vi "Write Y.vi"(8 "error in (no error)":errorcluster, 10 "Y":dbl[](array[numeric]), 11 "Y (1Ch) in":refnum<class "Y (1 Ch).lvclass">) -> (0 "error out":errorcluster, 3 "Y (1Ch) out":refnum<class "Y (1 Ch).lvclass">)   [LabVIEW 2017, in "Y (1 Ch).lvclass"]
uses:
  <vilib>/addons/_NISVFA/_Shared subVIs/Data Objects/Y (DBL)/Y (1 Ch).lvclass
  <vilib>/addons/_NISVFA/_Shared subVIs/Data Objects/Y (DBL)/Y (1 Ch).lvclass/Y (1 Ch).ctl
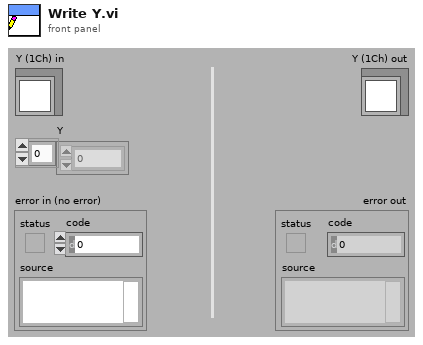
[diagram p1: front panel]
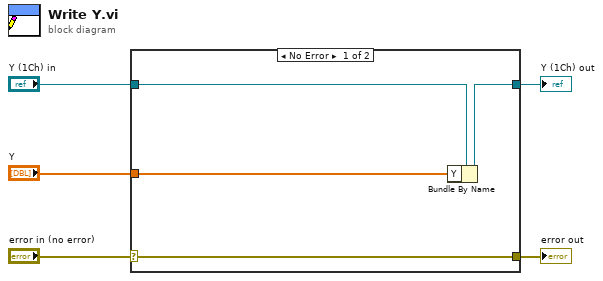
[diagram p0: block diagram]
diagram:
  n1 = case shown="No Error" "error in (no error)" {
    selector: "error in (no error)" -> [w9 w10]
    tunnel: [w9 w10] -> w4
    tunnel: [w6 w11] -> w2
    tunnel: "Y (1Ch) in" -> [w8 w11]
    tunnel: "Y" -> [w7 _]
    frame No Error {
      n2 = Bundle By Name(cluster=w8, "Y"=w7) -> (w6:refnum<class "Y (1 Ch).lvclass">)
    }
    frame Error {
    }
  }
  "error out" <- w4
  "Y (1Ch) out" <- w2
